vi "Write channel spctra (index).vi"(8 "error in (no error)":errorcluster, 10 "channel spectra (index DUT)":i32, 11 "OSA300 in":refnum<class "OSA300.lvclass">) -> (0 "error out":errorcluster, 3 "OSA300 out":refnum<class "OSA300.lvclass">)   [LabVIEW 2010, in "OSA300.lvclass"]
uses:
  OSA300.lvclass
  OSA300.lvclass/OSA300.ctl
  OSA20X_misc.lvlib
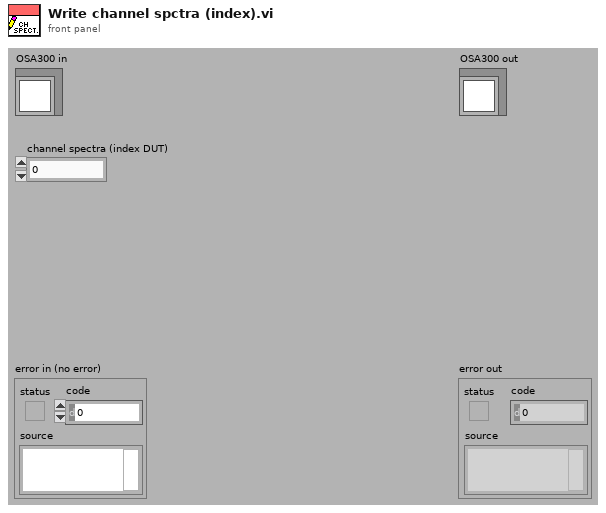
[diagram p1: front panel]
types:
  T1 = cluster{"waveMin (cm-1)":i32, "waveMax (cm-1)":i32, "gain":i32, "offset":i32, "damper available":bool, "damper active":bool}[]
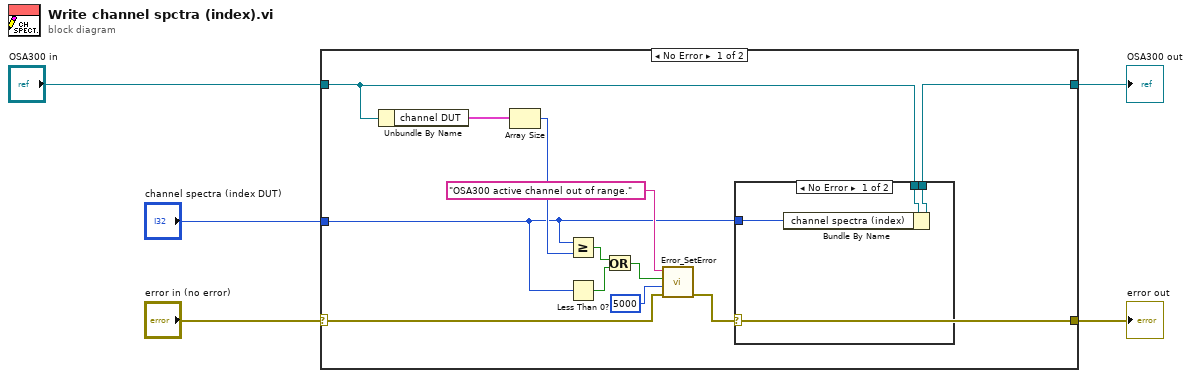
[diagram p0: block diagram]
diagram:
  n1 = case shown="No Error" "error in (no error)" {
    selector: "error in (no error)" -> [w15 w23]
    tunnel: [w7 w23] -> w4
    tunnel: [w17 w22] -> w3
    tunnel: "OSA300 in" -> [w6 w22]
    tunnel: "channel spectra (index DUT)" -> [w8 _]
    frame No Error {
      n2 = Unbundle By Name(w6) -> ("channel DUT"=w16:T1)
      n3 = Array Size(array=w16) -> (size(s)=w14:i32)
      n4 = Greater Or Equal?(x=w8, y=w14) -> (x >= y?=w13:bool)
      n5 = Less Than 0?(x=w8) -> (x < 0?=w11:bool)
      n6 = Or(x=w13, y=w11) -> (x .or. y?=w12:bool)
      n7 = call "Error_SetError.vi"("error in"=w15, "code(5000)"=5000, "status (true)"=w12, "source(\"\")"="OSA300 active channel out of range." ("source(\"\")")) -> ("error out"=w7:errorcluster)  [unwired: 3 in]
      n8 = case shown="No Error" w7 {
        tunnel: [w20 w21] -> w17
        tunnel: w6 -> [w19 w21]
        tunnel: w8 -> [w18 _]
        frame No Error {
          n9 = Bundle By Name(cluster=w19, "channel spectra (index)"=w18) -> (w20:refnum<class "OSA300.lvclass">)
        }
        frame Error {
        }
      }
    }
    frame Error {
    }
  }
  "error out" <- w4
  "OSA300 out" <- w3
